vi "Is Empty Cluster.vi"(1 "Deserialized JSON Data":variant) -> (0 "Empty Cluster?":bool)   [LabVIEW 2019, in "JKI JSON Serialization.lvlib"]
doc: "JKI JSON 1.1.10.37\nTomi Maila - JKI\nCopyright (c) 2017, JKI"
uses:
  JKI JSON Serialization.lvlib
  user.lib/_OpenG.lib/lvdata/lvdata.llb/Array of VData to VCluster__ogtk.vi
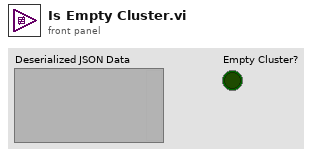
[diagram p1: front panel]
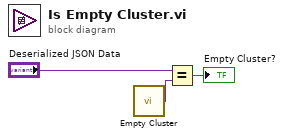
[diagram p0: block diagram]
diagram:
  n1 = call "Empty Cluster.vi"() -> ("Empty Cluster"=w2:variant)
  n2 = Equal?(x="Deserialized JSON Data", y=w2) -> (x = y?=→"Empty Cluster?":bool)
